vi "全局 地雷数组.vi"() -> ()   [LabVIEW 2017]
panel:
  out "地雷":i16[][](array[numeric])
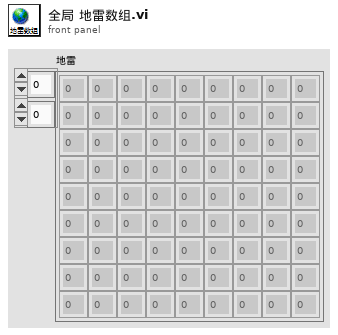
[diagram p1: front panel]
diagram:
